vi "Day04-01_변수.vi"() -> ()   [LabVIEW 2021]
panel:
  in  "숫자형 2":dbl
  in  "숫자형":dbl
  in  "정지 2":bool
  in  "정지":bool
  # "누를 때 스위치"
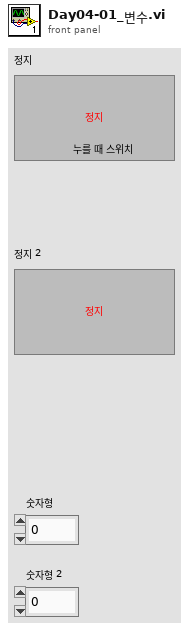
[diagram p1: front panel]
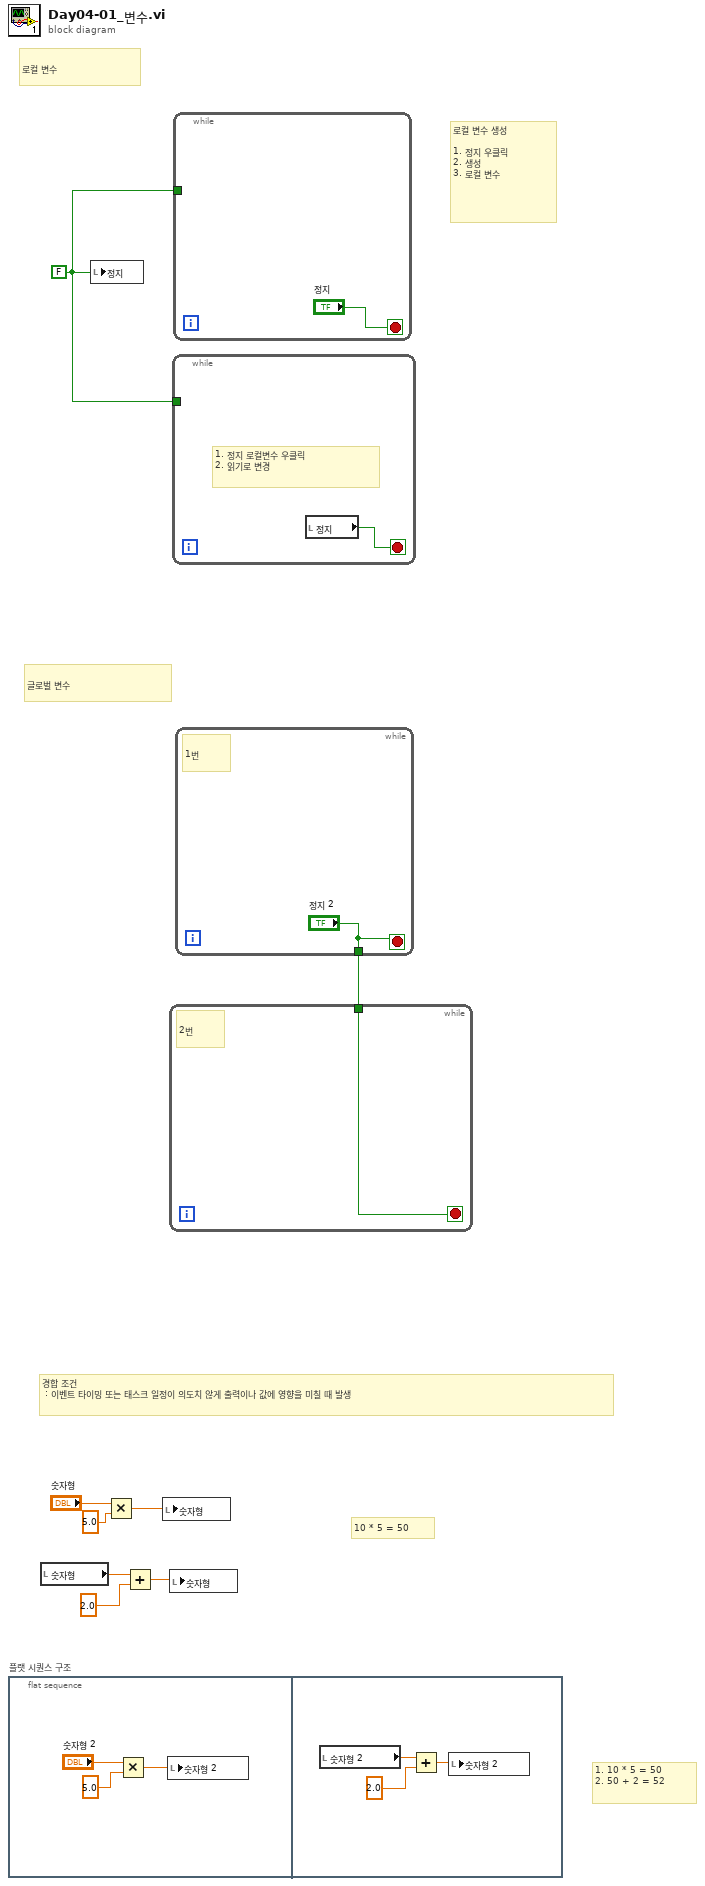
[diagram p0: block diagram]
diagram:
  w8 = FALSE
  # "1. 10 * 5 = 50\n2. 50 + 2 = 52"
  # "10 * 5 = 50"
  # "경합 조건\n : 이벤트 타이밍 또는 태스크 일정이 의도치 않게 출력이나 값에 영향을 미칠 때 발생"
  # "글로벌 변수"
  # "로컬 변수 생성\n\n1. 정지 우클릭\n2. 생성\n3. 로컬 변수"
  # "로컬 변수"
  n1 = flat-sequence "플랫 시퀀스 구조" {
    frame #0 {
      n2 = Multiply(x="숫자형 2", y=5.0) -> (x*y=w11:dbl)
      n3 = local write "숫자형 2"(w11) -> ()
    }
    frame #1 {
      n4 = local read "숫자형 2"() -> (w12:dbl)
      n5 = Add(x=w12, y=2.0) -> (x+y=w14:dbl)
      n6 = local write "숫자형 2"(w14) -> ()
    }
  }
  n7 = local read "숫자형"() -> (w3:dbl)
  n8 = local write "정지"(w8) -> ()
  n9 = Multiply(x="숫자형", y=5.0) -> (x*y=w4:dbl)
  n10 = Add(x=w3, y=2.0) -> (x+y=w1:dbl)
  n11 = local write "숫자형"(w4) -> ()
  n12 = local write "숫자형"(w1) -> ()
  n13 = while {
    tunnel: w8 -> [_]
    stop <- w15 stop-if-true
    # "1. 정지 로컬변수 우클릭\n2. 읽기로 변경"
    n14 = local read "정지"() -> (w15:bool)
  }
  n15 = while {
    tunnel: w8 -> [_]
    stop <- "정지" stop-if-true
  }
  n16 = while {
    tunnel: ["정지 2"] -> w7
    stop <- "정지 2" stop-if-true
    # "1번"
  }
  n17 = while {
    tunnel: w7 -> [w18]
    stop <- w18 stop-if-true
    # "2번"
  }
